vi "test--check_corner_islands.vi"() -> ()   [LabVIEW 2020, in "core.lvlib"]
uses:
  core.lvlib
  core_data/chess_square--chess notation.ctl
  core_data/file--enum.ctl
  core_data/rank--enum.ctl
  core_data/chessboard_index.ctl
  check_island.vi
  check_head_is_neighbour.vi
  get_chessboard_square.vi
  get all unexplored neighbours.vi
  PTRL/timing_utilities/timing_utilities.lvlib
  core_data/core_data.lvlib
panel:
  out "corner square that starts an island (chess notation)":T1
  out "corner square that starts an island (chessboard index)":T4
  out "T = a corner island was found":bool
  in  "head":T1
  out "test input 1":bool[][](array[boolean])=[[FALSE, TRUE, TRUE, TRUE, TRUE, TRUE, TRUE, TRUE], [TRUE, TRUE, TRUE, TRUE, TRUE, TRUE, TRUE, TRUE], [TRUE, FALSE, TRUE, TRUE, TRUE, TRUE, TRUE, TRUE], [TRUE, TRUE, TRUE, TRUE, TRUE, TRUE, TRUE, TRUE], [TRUE, TRUE, TRUE, TRUE, TRUE, TRUE, TRUE, TRUE], [TRUE, TRUE, TRUE, TRUE, TRUE, TRUE, TRUE, TRUE], [TRUE, TRUE, TRUE, TRUE, TRUE, TRUE, TRUE, TRUE], [TRUE, TRUE, TRUE, TRUE, TRUE, TRUE, TRUE, TRUE]]
  in  "chessboard (test input)":bool[][](array[boolean])=[[FALSE, TRUE, TRUE, TRUE, TRUE, TRUE, TRUE, TRUE], [TRUE, TRUE, TRUE, TRUE, TRUE, TRUE, TRUE, TRUE], [TRUE, FALSE, TRUE, TRUE, TRUE, TRUE, TRUE, TRUE], [TRUE, TRUE, TRUE, TRUE, TRUE, TRUE, TRUE, TRUE], [TRUE, TRUE, TRUE, TRUE, TRUE, TRUE, TRUE, TRUE], [TRUE, TRUE, TRUE, TRUE, TRUE, TRUE, TRUE, TRUE], [TRUE, TRUE, TRUE, TRUE, TRUE, TRUE, TRUE, TRUE], [TRUE, TRUE, TRUE, TRUE, TRUE, TRUE, TRUE, TRUE]] caption="Chessboard"
  # "Outputs"
  # "Inputs"
  # "8"
  # "7"
  # "6"
  # "5"
  # "4"
  # "3"
  # "2"
  # "1"
  # "a"
  # "b"
  # "c"
  # "d"
  # "e"
  # "f"
  # "g"
  # "h"
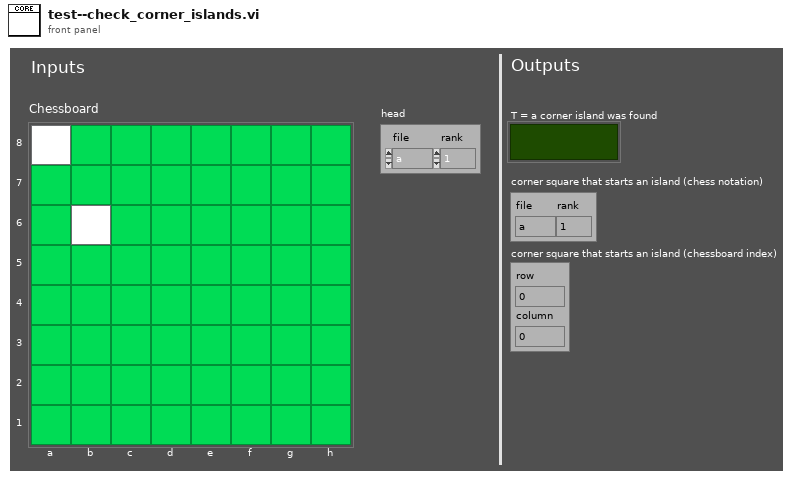
[diagram p1: front panel]
types:
  T1 = typedef "core.lvlib/core_data.lvlib/chess_square--chess notation.ctl" = cluster{"file":T2, "rank":T3}
  T2 = typedef "core.lvlib/core_data.lvlib/file--enum.ctl" = enum16{"a", "b", "c", "d", "e", "f", "g", "h"}
  T3 = typedef "core.lvlib/core_data.lvlib/rank--enum.ctl" = enum16{"1", "2", "3", "4", "5", "6", "7", "8"}
  T4 = typedef "core.lvlib/core_data.lvlib/chessboard_index.ctl" = cluster{"row":u8, "column":u8}
  T5 = typedef "core.lvlib/core_data.lvlib/tour_in_progress.ctl" = cluster{"start_time":timestamp, "tour":T4[], "no. of moves forward":u64, "no. of moves backward":u64}
  T6 = typedef "core.lvlib/core_data.lvlib/chess_square.ctl" = cluster{"Explored?":bool, "neighbouring_squares":T7[]}
  T7 = typedef "core.lvlib/core_data.lvlib/neighbour_square.ctl" = cluster{"row":u8, "column":u8, "exhausted?":bool}
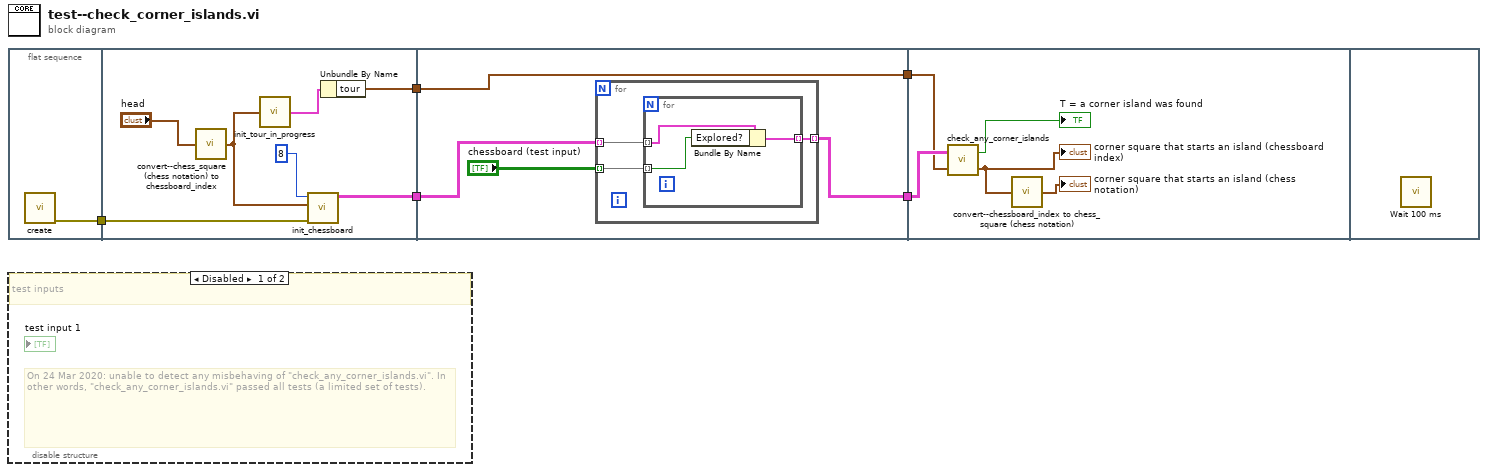
[diagram p0: block diagram]
diagram:
  n1 = flat-sequence {
    tunnel: [w6] -> w3
    tunnel: [w10] -> w5
    tunnel: w3 -> [w9]
    tunnel: [w7] -> w1
    tunnel: w5 -> [w15]
    tunnel: [w16] -> w4
    tunnel: [w14] -> w2
    tunnel: w1 -> [w14]
    tunnel: w4 -> [w28]
    tunnel: w2 -> [w24]
    frame #0 {
      n2 = call "create.vi"() -> ("error out"=w6:errorcluster)  [unwired: 11 in]
    }
    frame #1 {
      n3 = call "convert--chess_square (chess notation) to chessboard_index.vi"("chess_square (chess notation)"="head") -> ("chessboard_index"=w11:T4)
      n4 = call "init_tour_in_progress.vi"("starting_square"=w11) -> ("blank_tour_in_progress"=w8:T5)
      n5 = call "init_chessboard.vi"("error in (no error)"=w9, "starting_square"=w11, "chessboard_size"=u8 8) -> ("chessboard (populated)"=w10:T6[][])  [unwired: 7 in, 1 out]
      n6 = Unbundle By Name(w8) -> ("tour"=w7:T4[])
    }
    frame #2 {
      n7 = for {
        tunnel: "chessboard (test input)" -> [w19] mode=indexing
        tunnel: w15 -> [w20] mode=indexing
        tunnel: [w18] -> w16 mode=indexing
        n8 = for {
          tunnel: w20 -> [w23] mode=indexing
          tunnel: w19 -> [w22] mode=indexing
          tunnel: [w21] -> w18 mode=indexing
          n9 = Bundle By Name(cluster=w23, "Explored?"=w22) -> (w21:T6)
        }
      }
    }
    frame #3 {
      n10 = call "check_any_corner_islands.vi"("tour_in_progress"=w24, "chessboard"=w28) -> ("corner square that starts an island"=w26:T4, "T = a corner island was found"=→"T = a corner island was found":bool)
      "corner square that starts an island (chessboard index)" <- w26
      n11 = call "convert--chessboard_index to chess_square (chess notation).vi"("chessboard_index"=w26) -> ("chess_square (chess notation)"=→"corner square that starts an island (chess notation)":T1)
    }
    frame #4 {
      n12 = call "Wait 100 ms.vi"() -> ()  [unwired: 11 in, 1 out]
    }
  }
  n13 = disable-structure shown="Disabled" {
    frame Disabled {
      # "On 24 Mar 2020: unable to detect any misbehaving of \"check_any_corner_islands.vi\". In other words, \"check_any_corner_islands.vi\" passed all tests (a limited set of tests)."
      # "test inputs"
    }
    frame Enabled {
    }
  }
